vi "analog geneate signal.vi"() -> ()   [LabVIEW 2014]
uses:
  <vilib>/express/express arith-compare/Formula/XNode/ExpressFormulaBlockNode.xnode
panel:
  in  "VARS":dbl(slide) scale=7.5..20.0
  in  "stop":bool
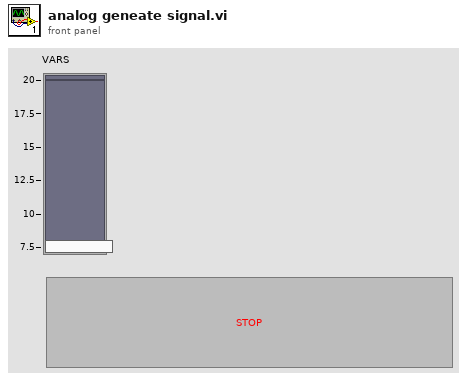
[diagram p1: front panel]
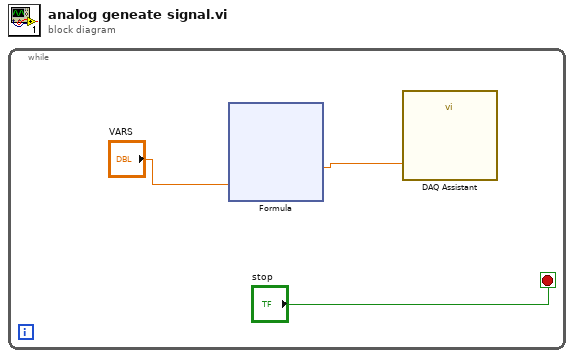
[diagram p0: block diagram]
diagram:
  n1 = while {
    stop <- "stop" stop-if-true
    n2 = xnode "Formula"("X"="VARS") -> ("Result"=w1:dbl)  [unwired: 1 in, 1 out]
    n3 = call "DAQ Assistant"("data"=w1) -> ()  [unwired: 17 in, 2 out]
  }
